vi "Launch Start Actors.vi"(8 "error in (no error)":errorcluster, 11 "CS++StartActor in":refnum<class "CS++StartActor.lvclass">) -> (0 "error out":errorcluster, 3 "CS++StartActor out":refnum<class "CS++StartActor.lvclass">)   [LabVIEW 2016, in "CS++StartActor.lvlib" / "CS++StartActor.lvclass"]
doc: "Launch Start Actors."
uses:
  CS++StartActor.lvclass
  C:/User/Brand/LVP/CSPP/Packages/CSPP_Core/Actors/CS++BaseActor/CS++BaseActor.lvclass
  C:/Program Files (x86)/National Instruments/LabVIEW 2016/vi.lib/ActorFramework/Actor/Actor.lvclass
  CS++BaseActor/CS++BaseActor.lvclass/CS++BaseActor.ctl
  CS++StartActor.lvclass/CS++StartActor.ctl
  CS++BaseActor Messages/Open Actor Core FP Msg/Open Actor Core FP Msg.lvclass/Open Actor Core FP Msg.ctl
  <vilib>/ActorFramework/Message Enqueuer/Message Enqueuer.lvclass/Message Enqueuer.ctl
  <vilib>/ActorFramework/Message Enqueuer/Enqueue.vi
  CS++BaseActor/CS++BaseActor.lvclass
  CS++BaseActor Messages/Open Actor Core FP Msg/Open Actor Core FP Msg.lvclass
  C:/Program Files (x86)/National Instruments/LabVIEW 2016/vi.lib/ActorFramework/Message/Message.lvclass
  <vilib>/ActorFramework/Message Priority Queue/Priority Enqueue.vi
  Classes/CS++BaseClasses/Factory/CS++Factory.lvclass
  <vilib>/ActorFramework/Actor/Actor.lvclass
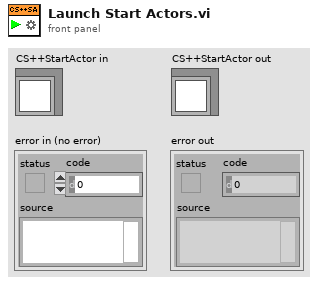
[diagram p1: front panel]
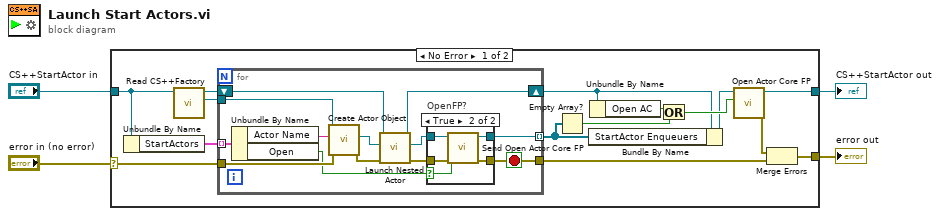
[diagram p0: block diagram]
diagram:
  n1 = case shown="No Error" "error in (no error)" {
    selector: "error in (no error)" -> [w18 w41]
    tunnel: [w11 w41] -> w3
    tunnel: [w12 w40] -> w1
    tunnel: "CS++StartActor in" -> [w6 w40]
    frame No Error {
      n2 = Unbundle By Name(w6) -> ("StartActors"=w19:cluster{"Actor Name":string, "Open":bool}[])
      n3 = call "Read CS++Factory.vi"("CS++BaseActor in"=w6) -> ("CS++Factory"=w16:refnum<class "CS++Factory.lvclass">, "CS++BaseActor out"=w7:refnum<class "CS++StartActor.lvclass">)  [unwired: 8 in, 1 out]
      n4 = for {
        tunnel: w19 -> [w29] mode=indexing
        tunnel: w16 -> [w32]
        tunnel: w18 -> [w31]
        tunnel: [w26] -> w17
        tunnel: [w24] -> w8 mode=indexing
        shift-right: [w20] -> w5
        shift-left: w7 -> [w21]
        stop <- w26 stop-if-true
        n5 = Unbundle By Name(w29) -> ("Actor Name"=w28:string, "Open"=w23:bool)
        n6 = call "Create Actor Object.vi"("error in (no error)"=w31, "Object Name"=w28, "CS++Factory in"=w32) -> ("error out"=w30:errorcluster, "CS++BaseActor"=w22:refnum<class "CS++BaseActor.lvclass">)  [unwired: 5 in, 2 out]
        n7 = call <vilib>:"Launch Nested Actor.vi"("error in (no error)"=w30, "Nested Actor"=w22, "Caller Actor in"=w21) -> ("error out"=w27:errorcluster, "Nested Actor's Enqueuer"=w25:refnum<class "Message Enqueuer.lvclass">, "Caller Actor out"=w20:refnum<class "CS++StartActor.lvclass">)  [unwired: 6 in]
        n8 = case "OpenFP?" shown="True" w23 {
          selector: w23 -> [_ w35]
          tunnel: w27 -> [w33 w39]
          tunnel: [w33 w38] -> w26
          tunnel: w25 -> [w34 w37]
          tunnel: [w34 w36] -> w24
          frame False {
          }
          frame True {
            n9 = call "Send Open Actor Core FP.vi"("error in (no error)"=w39, "Open FP (F)"=w35, "Message Enqueuer"=w37) -> ("error out"=w38:errorcluster, "Message Enqueuer out"=w36:refnum<class "Message Enqueuer.lvclass">)  [unwired: 7 in]
          }
        }
      }
      n10 = Empty Array?(array=w8) -> (empty?=w9:bool)
      n11 = Bundle By Name(cluster=w5, "StartActor Enqueuers"=w8) -> (w13:refnum<class "CS++StartActor.lvclass">)
      n12 = Unbundle By Name(w5) -> ("Open AC"=w15:bool)
      n13 = Or(x=w15, y=w9) -> (x .or. y?=w14:bool)
      n14 = call "Open Actor Core FP.vi"("Open FP (F)"=w14, "CS++BaseActor in"=w13) -> ("error out"=w10:errorcluster, "CS++BaseActor out"=w12:refnum<class "CS++StartActor.lvclass">)  [unwired: 8 in]
      n15 = Merge Errors(w10, w17) -> (w11:errorcluster)
    }
    frame Error {
    }
  }
  "error out" <- w3
  "CS++StartActor out" <- w1
